vi "Wizard Default Path.vi"(2 "Mode":enum16{"Error List"}(ring)) -> (0 "Path":path)   [LabVIEW 2014]
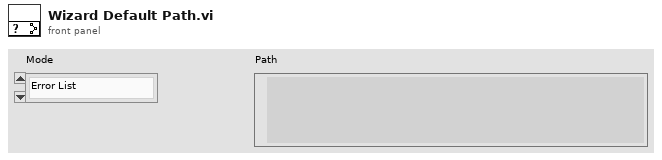
[diagram p1: front panel]
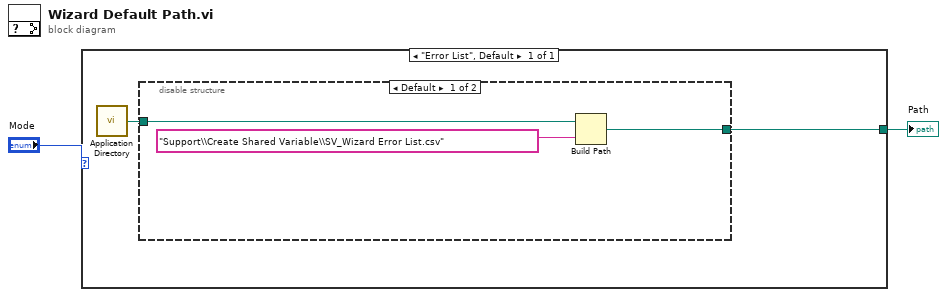
[diagram p0: block diagram]
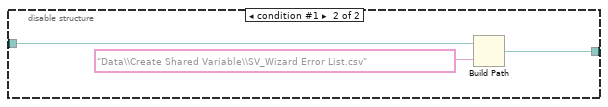
[diagram p2: hidden frame]
diagram:
  n1 = case shown="\"Error List\", Default" "Mode" {
    tunnel: [w3] -> w1
    frame "Error List", Default {
      n2 = call <vilib>:"Application Directory.vi"() -> ("Application Directory"=w4:path)
      n3 = disable-structure shown="Default" {
        disable-tunnel: w4 -> [w7 w9]
        disable-tunnel: [w5 w8] -> w3
        frame condition #0 (active) {
          n4 = Build Path(base path=w7, name or relative path="Support\\Create Shared Variable\\SV_Wizard Error List.csv") -> (appended path=w5:path)
        }
        frame condition #1 {
          n5 = Build Path(base path=w9, name or relative path="Data\\Create Shared Variable\\SV_Wizard Error List.csv") -> (appended path=w8:path)
        }
      }
    }
  }
  "Path" <- w1
